vi "Find.vi"(7 "default":refnum<class "Buffer Converter.lvclass">, 8 "error in (no error)":errorcluster, 11 "Components":refnum<class "Component.lvclass">[](array[class])) -> (0 "error out":errorcluster, 1 "component name":string, 2 "found?":bool, 3 "Buffer Converter":refnum<class "Buffer Converter.lvclass">)   [LabVIEW 2019, in "DSF Core.lvlib" / "Buffer Converter.lvclass"]
uses:
  Buffer Converter.lvclass
  Component/Component.lvclass
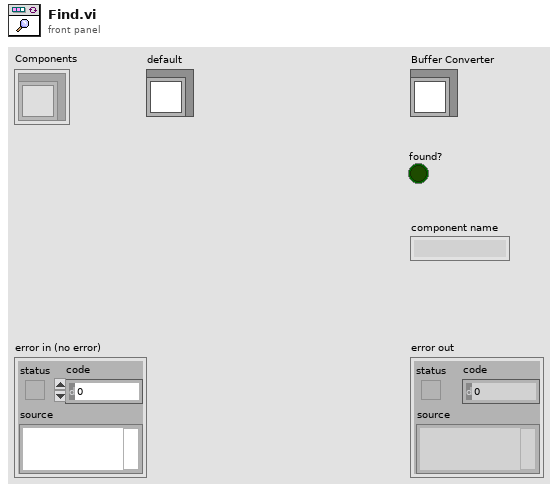
[diagram p1: front panel]
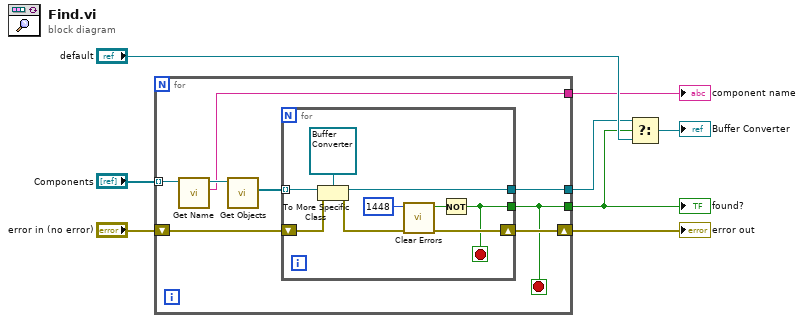
[diagram p0: block diagram]
diagram:
  n1 = for {
    tunnel: "Components" -> [w11] mode=indexing
    tunnel: [w15] -> w3
    tunnel: [w12] -> w4
    shift-right: [w14] -> w5
    shift-left: "error in (no error)" -> [w16]
    tunnel: [w9] -> w1
    stop <- w12 stop-if-true
    n2 = call "Get Name.vi"("Component in"=w11) -> ("name"=w9:string, "Component out"=w10:refnum<class "Component.lvclass">)  [unwired: 9 in]
    n3 = call "Get Objects.vi"("Component in"=w10) -> ("objects"=w13:refnum<class>[])  [unwired: 9 in, 1 out]
    n4 = for {
      tunnel: w13 -> [w25] mode=indexing
      shift-right: [w22] -> w14
      shift-left: w16 -> [w21]
      tunnel: [w19] -> w12
      tunnel: [w18] -> w15
      stop <- w19 stop-if-true
      n5 = To More Specific Class(target class=refnum<class "Buffer Converter.lvclass"> refnum ("default"), reference=w25, error in=w21) -> (specific class reference=w18:refnum<class "Buffer Converter.lvclass">, error out=w23:errorcluster)
      n6 = call <vilib>:"Clear Errors.vi"("error in (no error)"=w23, "specific error code to clear (0: all)"=1448) -> ("error out"=w22:errorcluster, "specific error cleared?"=w20:bool)  [unwired: 4 in]
      n7 = Not(x=w20) -> (.not. x?=w19:bool)
    }
  }
  "error out" <- w5
  "found?" <- w4
  "component name" <- w1
  n8 = Select(t=w3, s=w4, f="default") -> (s? t:f=→"Buffer Converter":refnum<class "Buffer Converter.lvclass">)
